vi "Count.vi"() -> ()   [LabVIEW 2011]
panel:
  out "x-y":u32
  out "x-y":u32
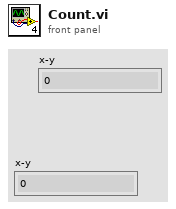
[diagram p1: front panel]
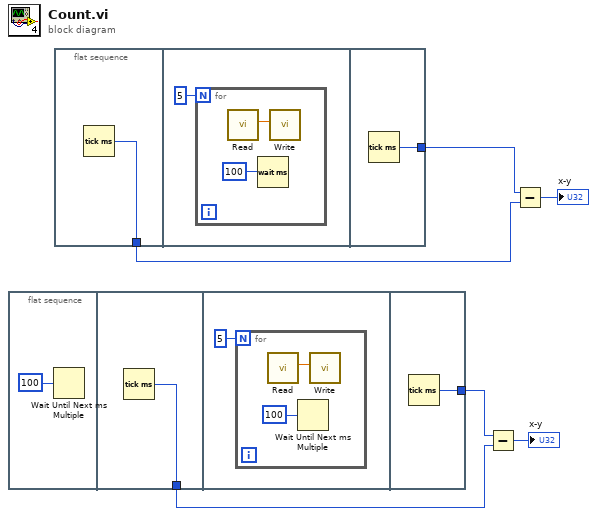
[diagram p0: block diagram]
diagram:
  n1 = flat-sequence {
    tunnel: [w8] -> w5
    tunnel: [w12] -> w6
    frame #0 {
      n2 = Wait Until Next ms Multiple(millisecond multiple=u32 100) -> ()  [unwired: 1 out]
    }
    frame #1 {
      n3 = Tick Count (ms)() -> (millisecond timer value=w8:u32)
    }
    frame #2 {
      n4 = for {
        N: 5 -> [_]
        n5 = call "Read.vi"() -> ("Numeric"=w11:dbl)  [unwired: 11 in]
        n6 = Wait Until Next ms Multiple(millisecond multiple=u32 100) -> ()  [unwired: 1 out]
        n7 = call "Write.vi"("Numeric"=w11) -> ()  [unwired: 11 in]
      }
    }
    frame #3 {
      n8 = Tick Count (ms)() -> (millisecond timer value=w12:u32)
    }
  }
  n9 = flat-sequence {
    tunnel: [w13] -> w2
    tunnel: [w17] -> w1
    frame #0 {
      n10 = Tick Count (ms)() -> (millisecond timer value=w13:u32)
    }
    frame #1 {
      n11 = for {
        N: 5 -> [_]
        n12 = call "Read.vi"() -> ("Numeric"=w16:dbl)  [unwired: 11 in]
        n13 = Wait (ms)(milliseconds to wait=u32 100 ("millisecond multiple")) -> ()  [unwired: 1 out]
        n14 = call "Write.vi"("Numeric"=w16) -> ()  [unwired: 11 in]
      }
    }
    frame #2 {
      n15 = Tick Count (ms)() -> (millisecond timer value=w17:u32)
    }
  }
  n16 = Subtract(x=w6, y=w5) -> (x-y=→"x-y":u32)
  n17 = Subtract(x=w1, y=w2) -> (x-y=→"x-y":u32)
